vi "Core.vi"(8 "error in (no error)":errorcluster, 10 "Actor in":refnum<class "Actor.lvclass">, 11 "Open File Msg in":refnum<class "Open File Msg.lvclass">) -> (0 "error out":errorcluster, 1 "Data":refnum<class "Data.lvclass">, 2 "Actor out":refnum<class "Actor.lvclass">, 3 "Open File Msg out":refnum<class "Open File Msg.lvclass">)   [LabVIEW 2020, in "File Writer.lvlib" / "Open File Msg.lvclass"]
doc: "Core of the Reponse Msg. Put the active code here.\n\nThe defaul implementation does nothing."
uses:
  Open File Msg.lvclass
  PPL/HDH.Data.Generic.lvlibp/Data.lvclass
  PPL/HDH.Actor Framework.Core.Actor.lvlibp/1abvi3w/vi.lib/ActorFramework/Actor/Actor.lvclass
  File Writer/File Writer.lvclass
  C:/Current projects/WS/PPL/HDH.Actor Framework.Core.Actor.lvlibp/1abvi3w/vi.lib/ActorFramework/Actor/Actor.lvclass
  Open File Msg.lvclass/Open File Msg.ctl
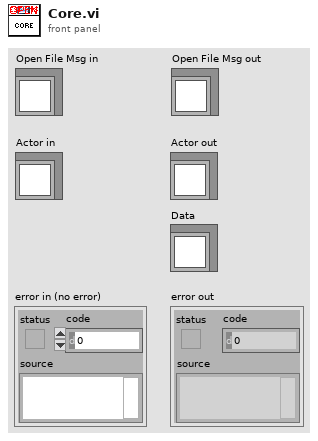
[diagram p1: front panel]
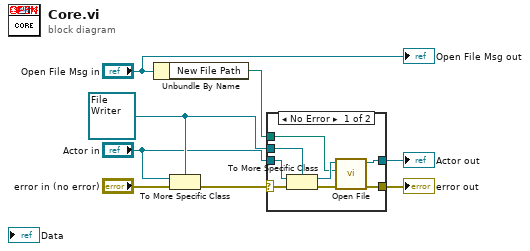
[diagram p0: block diagram]
diagram:
  w7 = refnum<class "File Writer.lvclass"> refnum ("Actor in")
  n1 = Unbundle By Name("Open File Msg in") -> ("New File Path"=w6:path)
  n2 = To More Specific Class(target class=w7, reference="Actor in", error in="error in (no error)") -> (error out=w8:errorcluster)  [unwired: 1 out]
  n3 = case shown="No Error" w8 {
    selector: w8 -> [w10 w18]
    tunnel: [w16 w18] -> w2
    tunnel: [w15 w17] -> w3
    tunnel: "Actor in" -> [w14 w17]
    tunnel: w7 -> [w13 _]
    tunnel: w6 -> [w11 _]
    frame No Error {
      n4 = To More Specific Class(target class=w13, reference=w14, error in=w10) -> (specific class reference=w12:refnum<class "File Writer.lvclass">, error out=w9:errorcluster)
      n5 = call "Open File.vi"("error in (no error)"=w9, "New File Path"=w11, "File Writer in"=w12) -> ("error out"=w16:errorcluster, "File Writer out"=w15:refnum<class "File Writer.lvclass">)  [unwired: 6 in, 1 out]
    }
    frame Error {
    }
  }
  "error out" <- w2
  "Actor out" <- w3
  "Open File Msg out" <- "Open File Msg in"
